vi "20151004 sensor+servo.vi"(0 "Serial Port":refnum<visa-resource-name>="COM10", 1 "Pulse Widths (uS)":u16[](array[numeric])=[1400, 1400, 1300, 1600, 1500, 1400, 1500, 1500, 1400, 1400, 1200, 1500] min=600 max=2400 step=100, 2 "Loop time":u32=100, 5 "Action(hardware)":T1(ring), 7 "Device Address":T2, 9 "Servo Channels":u8[](array[numeric])=[2, 3, 4, 5, 6, 7, 8, 9, 10, 11, 12, 13], 11 "error in (no error)":errorcluster) -> (4 "pitch":dbl, 6 "roll":dbl, 10 "Initialize OK?":bool=TRUE, 15 "Error Out":errorcluster)   [LabVIEW 2013]
uses:
  <vilib>/MakerHub/LINX/Public/Sensors/Accelerometer/MPU60X0/DeviceAddresses.ctl
  <vilib>/MakerHub/LINX/Public/Sensors/Motion/Servo/Servo Open N Channels.vi
  <vilib>/MakerHub/LINX/Public/Sensors/Motion/Servo/Servo Set Pulse Width N Channels.vi
  <vilib>/MakerHub/LINX/Public/Sensors/Motion/Servo/Servo Close N Channels.vi
  <vilib>/MakerHub/LINX/LMH-LINX.lvlib
  <vilib>/MakerHub/LINX/Public/Sensors/Motion/Servo/Servo.lvlib
  <vilib>/MakerHub/LINX/Public/Sensors/Accelerometer/MPU60X0/MPU60X0.lvlib
panel:
  out "Waveform Chart":T3(graph)
  # "up: CK"
  # "up: CK"
  # "up: CCK"
  # "up: CK"
  # "up: CK"
  # "up: CCK"
  # "up: CK"
  # "up: CK"
  # "up: CCK"
  # "up: CK"
  # "up: CK"
  # "up: CCK"
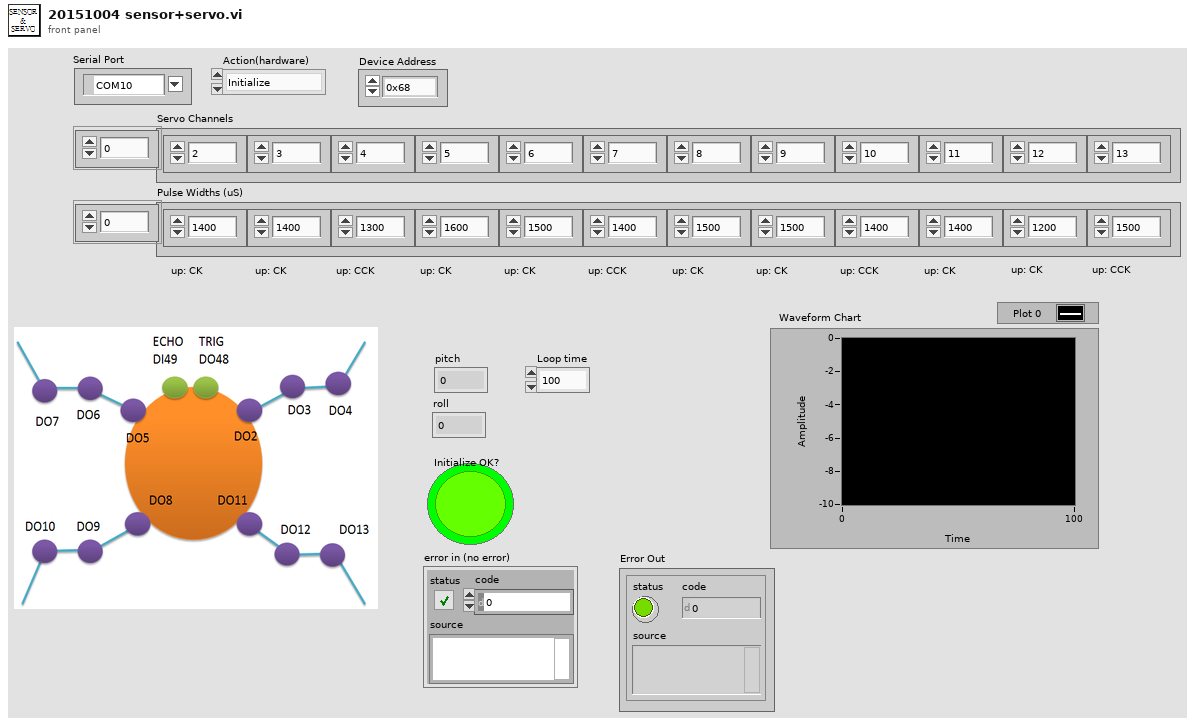
[diagram p1: front panel]
types:
  T1 = enum16{"Initialize", "Read acc & gyro", "Write servos", "Stop"}
  T2 = typedef "LMH-LINX.lvlib/MPU60X0.lvlib/DeviceAddresses.ctl" = enum16{"0x68", "0x69"}
  T3 = cluster{"pitch":dbl, "roll":dbl, "x_angle":dbl, "x_angle":dbl}
  T4 = typedef "LMH-LINX.lvlib/LINX Ref.ctl" = cluster{"Platform":T5, "Interface":T6, "LINX Device Config":T7}
  T5 = typedef "LMH-LINX.lvlib/Platform.ctl" = enum16{"LINX", "myRIO"}
  T6 = typedef "LMH-LINX.lvlib/Interface.ctl" = enum16{"Serial", "TCP"}
  T7 = typedef "LMH-LINX.lvlib/Device.lvlib/LINX Device Config.ctl" = cluster{"Interface":T6, "COM Port":refnum<visa-resource-name>, "TCP Configuration":T8, "Device Family":u8, "Device ID":u8, "Device Name":string, "TCP Ref":refnum<k5>, "Channels":T9}
  T8 = typedef "LMH-LINX.lvlib/Device.lvlib/TCP Config.ctl" = cluster{"IP Address":string, "Port":u16}
  T9 = typedef "LMH-LINX.lvlib/Channels.ctl" = cluster{"DI":u8[], "DO":u8[], "AI":u8[], "AO":u8[], "PWM":u8[], "QE":u8[], "UART":u8[], "I2C 2":u8[], "SPI":u8[], "CAN":u8[], "Servo":u8[], "AI Ref (V)":dbl, "AO Ref (V)":dbl, "AO Resolution (Bits)":u8}
  T10 = cluster{"X Axis":i16, "Y Axis":i16, "Z Axis":i16}
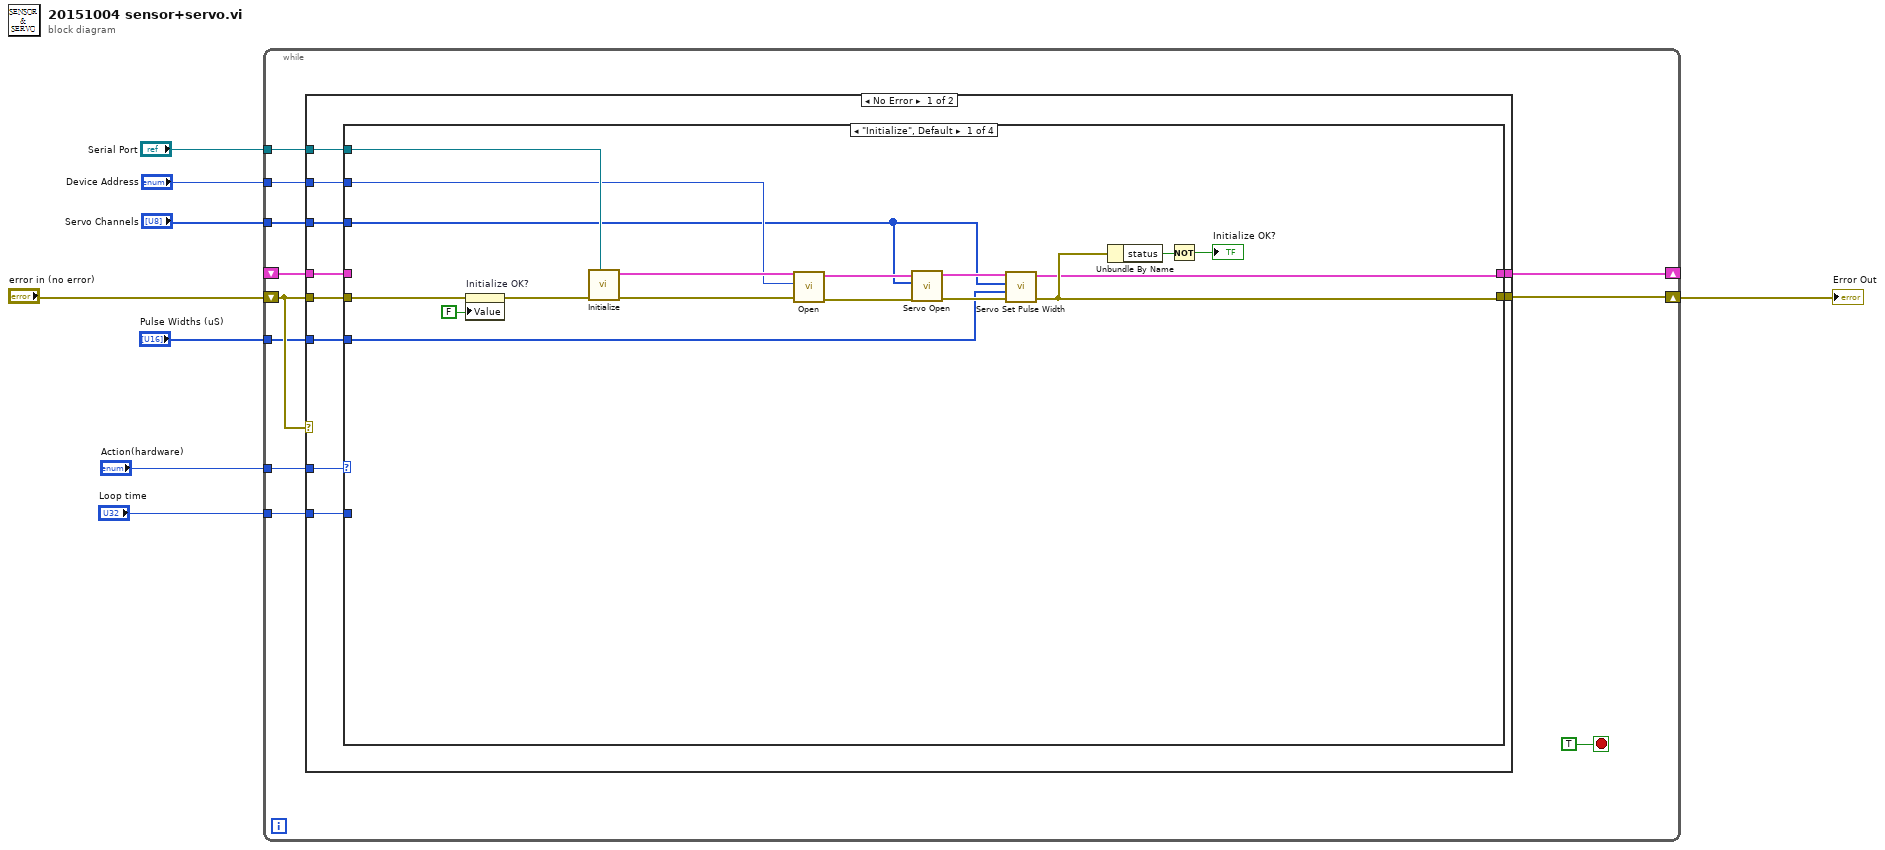
[diagram p0: block diagram]
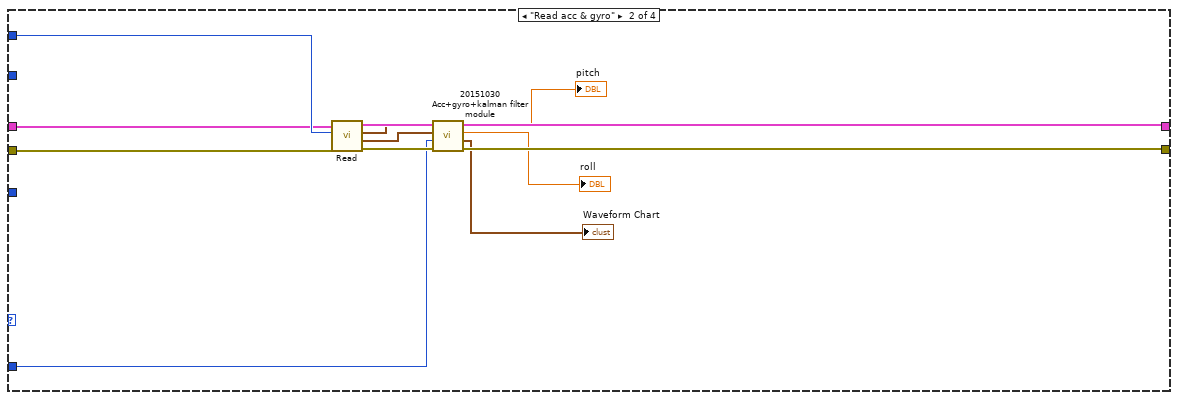
[diagram p2: hidden frame]
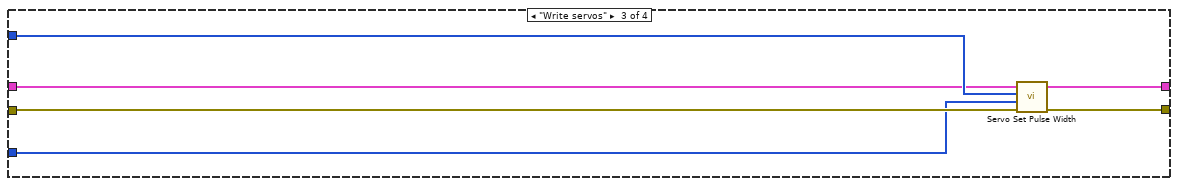
[diagram p3: hidden frame]
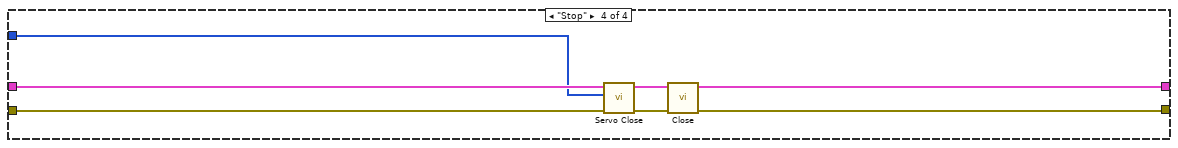
[diagram p4: hidden frame]
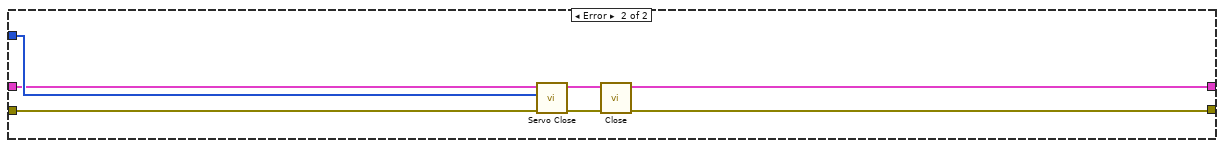
[diagram p5: hidden frame]
diagram:
  n1 = while {
    shift-right: [w19] -> w3
    shift-left: "error in (no error)" -> [w11]
    tunnel: "Servo Channels" -> [w17]
    shift-right: [w18] -> _
    shift-left: _ -> [w16]
    tunnel: "Device Address" -> [w15]
    tunnel: "Action(hardware)" -> [w14]
    tunnel: "Serial Port" -> [w13]
    tunnel: "Loop time" -> [w10]
    tunnel: "Pulse Widths (uS)" -> [w9]
    stop <- TRUE stop-if-true
    n2 = case shown="No Error" w11 {
      tunnel: [w29 w73] -> w19
      tunnel: [w28 w71] -> w18
      tunnel: w17 -> [w27 w74]
      tunnel: w16 -> [w26 w72]
      tunnel: w11 -> [w25 w75]
      tunnel: w15 -> [w24 _]
      tunnel: w14 -> [w23 _]
      tunnel: w13 -> [w22 _]
      tunnel: w10 -> [w21 _]
      tunnel: w9 -> [w20 _]
      frame No Error {
        n3 = case shown="\"Initialize\", Default" w23 {
          tunnel: [w34 w50 w63 w65] -> w29
          tunnel: [w32 w54 w62 w64] -> w28
          tunnel: w27 -> [w31 _ w61 w66]
          tunnel: w26 -> [_ w56 w60 w67]
          tunnel: w25 -> [w39 w55 w59 w68]
          tunnel: w24 -> [w37 w57 _ _]
          tunnel: w22 -> [w38 _ _ _]
          tunnel: w21 -> [_ w46 _ _]
          tunnel: w20 -> [w30 _ w58 _]
          frame "Initialize", Default {
            n4 = property on="Initialize OK?" class="Bool (strict)"(error in=w39, "Value"=FALSE ("Initialize OK?")) -> (error out=w40:errorcluster)  [unwired: 1 in, 1 out]
            n5 = call <vilib>:"Initialize.vi"("Serial Port"=w38, "Error In"=w40) -> ("Error Out"=w43:errorcluster, "LINX Ref"=w42:T4)  [unwired: 7 in, 1 out]
            n6 = call <vilib>:"Open.vi"("Error In"=w43, "Device Address"=w37, "LINX Resource"=w42) -> ("Error Out"=w45:errorcluster, "LINX Resource"=w44:T4)  [unwired: 7 in]
            n7 = call-poly <vilib>:"Servo Open.vi"("Error In"=w45, "Servo Channels"=w31, "LINX Resource"=w44) -> ("Error Out"=w34:errorcluster, "LINX Resource"=w33:T4)  [unwired: 7 in]
            n8 = call-poly <vilib>:"Servo Set Pulse Width.vi"("Pulse Widths (uS)"=w30, "Servo Channels"=w31, "LINX Resource"=w33) -> ("LINX Resource"=w32:T4)  [unwired: 7 in, 1 out]
            n9 = Unbundle By Name(w34) -> ("status"=w35:bool)
            n10 = Not(x=w35) -> (.not. x?=→"Initialize OK?":bool)
          }
          frame "Read acc & gyro" {
            n11 = call <vilib>:"Read.vi"("Error In"=w55, "Device Address"=w57, "LINX Resource"=w56) -> ("Error Out"=w53:errorcluster, "Gyro  Data"=w51:T10, "Acceleration Data"=w52:T10, "LINX Resource"=w54:T4)  [unwired: 4 in, 1 out]
            n12 = call "20151030 Acc+gyro+kalman filter module.vi"("error in (no error)"=w53, "Looptime"=w46, "Gyro  Data"=w51, "Acceleration Data"=w52) -> ("error out"=w50:errorcluster, "After Kalman filter"=→"Waveform Chart":T3, "roll"=→"roll":dbl, "pitch"=→"pitch":dbl)  [unwired: 4 in]
          }
          frame "Write servos" {
            n13 = call-poly <vilib>:"Servo Set Pulse Width.vi"("Error In"=w59, "Pulse Widths (uS)"=w58, "Servo Channels"=w61, "LINX Resource"=w60) -> ("Error Out"=w63:errorcluster, "LINX Resource"=w62:T4)  [unwired: 6 in]
          }
          frame "Stop" {
            n14 = call-poly <vilib>:"Servo Close.vi"("Error In"=w68, "Servo Channels"=w66, "LINX Resource"=w67) -> ("Error Out"=w70:errorcluster, "LINX Resource"=w69:T4)  [unwired: 7 in]
            n15 = call <vilib>:"Close.vi"("Error In"=w70, "LINX Resource"=w69) -> ("Error Out"=w65:errorcluster, "LINX Resource"=w64:T4)  [unwired: 8 in]
          }
        }
      }
      frame Error {
        n16 = call-poly <vilib>:"Servo Close.vi"("Error In"=w75, "Servo Channels"=w74, "LINX Resource"=w72) -> ("Error Out"=w77:errorcluster, "LINX Resource"=w76:T4)  [unwired: 7 in]
        n17 = call <vilib>:"Close.vi"("Error In"=w77, "LINX Resource"=w76) -> ("Error Out"=w73:errorcluster, "LINX Resource"=w71:T4)  [unwired: 8 in]
      }
    }
  }
  "Error Out" <- w3
